vi "DM65-Tutorial-2.vi"() -> ()   [LabVIEW 2020]
uses:
  C:/TwinCAT/AdsApi/.NET/v4.0.30319/TwinCAT.Ads.dll
  TwinCAT/AdsApi/.NET/v4.0.30319/TwinCAT.Ads.dll
panel:
  in  "stop":bool
  in  "start":bool
  out "box":bool
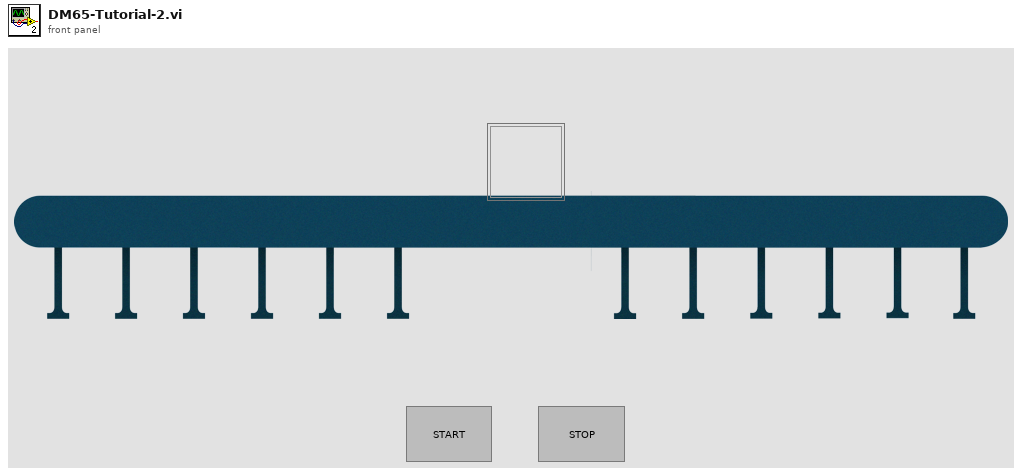
[diagram p1: front panel]
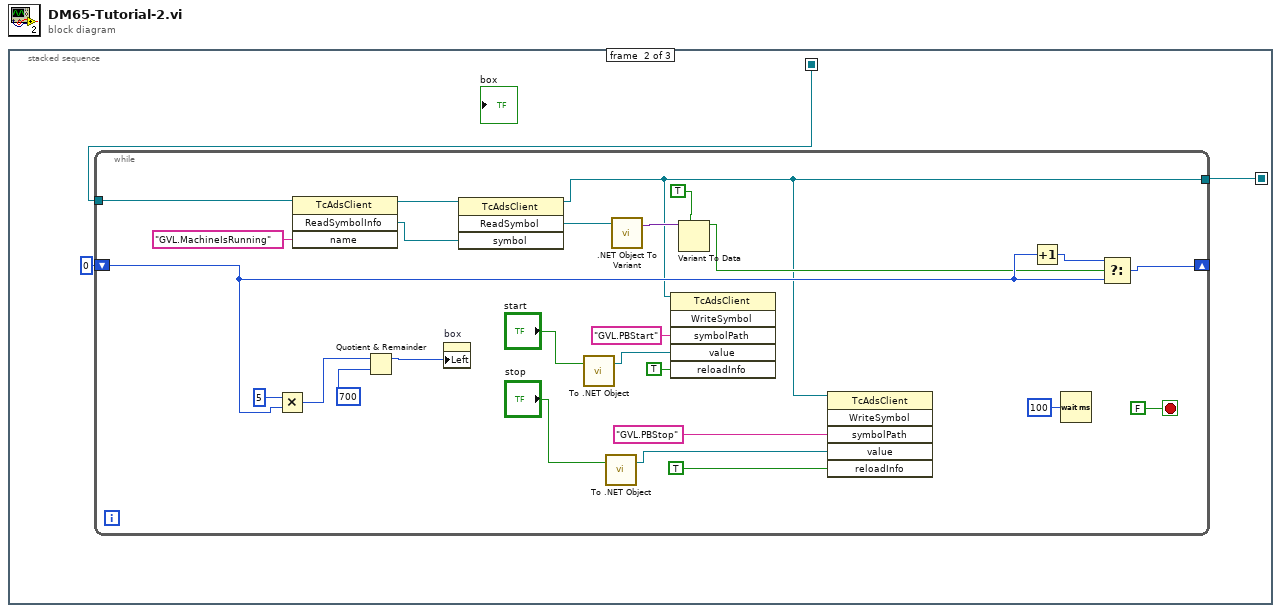
[diagram p0: block diagram]
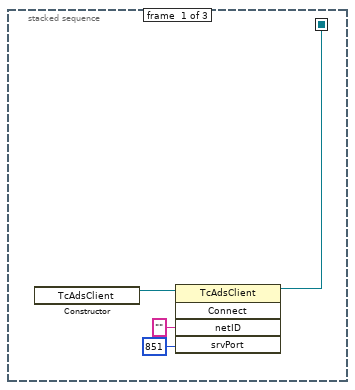
[diagram p2: hidden frame]
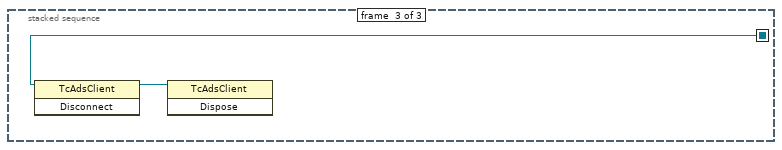
[diagram p3: hidden frame]
diagram:
  n1 = stacked-sequence {
    seq-local: [w1 _ _] -> [_ w6 _]
    seq-local: [_ w5 _] -> [_ _ w35]
    frame #0 {
      n2 = constructor class="TcAdsClient"() -> (reference out=w4:refnum<k24>)  [unwired: 3 in, 2 out]
      n3 = invoke class="TcAdsClient" method="Connect"(reference=w4, "netID"="", "srvPort"=851) -> (reference out=w1:refnum<k24>)  [unwired: 2 in, 4 out]
    }
    frame #1 {
      n4 = while {
        shift-right: [w29] -> _
        shift-left: 0 -> [w27]
        tunnel: w6 -> [w26]
        tunnel: [w8] -> w5
        stop <- FALSE stop-if-true
        n5 = Multiply(x=5, y=w27) -> (x*y=w31:i32)
        n6 = invoke class="TcAdsClient" method="ReadSymbolInfo"(reference=w26, "name"="GVL.MachineIsRunning") -> (reference out=w24:refnum<k24>, "ReadSymbolInfo"=w23:refnum<k24>)  [unwired: 2 in, 2 out]
        n7 = Quotient & Remainder(x=w31, y=700) -> (x-y*floor(x/y)=w17:i32)  [unwired: 1 out]
        n8 = property on="box" class="Bool (strict)"("Left"=w17) -> ()  [unwired: 2 in, 2 out]
        n9 = invoke class="TcAdsClient" method="ReadSymbol"(reference=w24, "symbol"=w23) -> (reference out=w8:refnum<k24>, "ReadSymbol"=w22:refnum<k24>)  [unwired: 2 in, 2 out]
        n10 = call <vilib>:"To .NET Object.vi"("anything"="start") -> (".NET object"=w14:refnum<k24>)  [unwired: 1 in, 1 out]
        n11 = call <vilib>:"To .NET Object.vi"("anything"="stop") -> (".NET object"=w11:refnum<k24>)  [unwired: 1 in, 1 out]
        n12 = call <vilib>:".NET Object To Variant.vi"(".NET object"=w22) -> ("variant"=w21:variant)  [unwired: 1 in, 1 out]
        n13 = invoke class="TcAdsClient" method="WriteSymbol"(reference=w8, "symbolPath"="GVL.PBStart", "value"=w14, "reloadInfo"=TRUE) -> ()  [unwired: 2 in, 6 out]
        n14 = Variant To Data(type=TRUE, Variant=w21) -> (data=w19:bool)  [unwired: 1 in, 1 out]
        n15 = invoke class="TcAdsClient" method="WriteSymbol"(reference=w8, "symbolPath"="GVL.PBStop", "value"=w11, "reloadInfo"=TRUE) -> ()  [unwired: 2 in, 6 out]
        n16 = Increment(x=w27) -> (x+1=w28:i32)
        n17 = Wait (ms)(milliseconds to wait=u32 100) -> ()  [unwired: 1 out]
        n18 = Select(t=w28, s=w19, f=w27) -> (s? t:f=w29:i32)
      }
    }
    frame #2 {
      n19 = invoke class="TcAdsClient" method="Disconnect"(reference=w35) -> (reference out=w34:refnum<k24>)  [unwired: 2 in, 2 out]
      n20 = invoke class="TcAdsClient" method="Dispose"(reference=w34) -> ()  [unwired: 2 in, 3 out]
    }
  }
